vi "PicRead.vi"() -> ()   [LabVIEW 2012]
panel:
  out "二维图片":picture
  in  "path to JPEG file":path caption="JPEG文件路径"
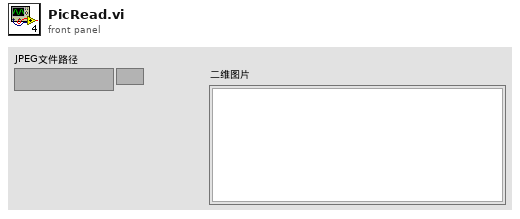
[diagram p1: front panel]
types:
  T1 = typedef "imagedata.ctl" = cluster{"image type":i32, "image depth":i32, "image":u8[], "mask":u8[], "colors":u32[], "Rectangle":cluster{"left":i16, "top":i16, "right":i16, "bottom":i16}}
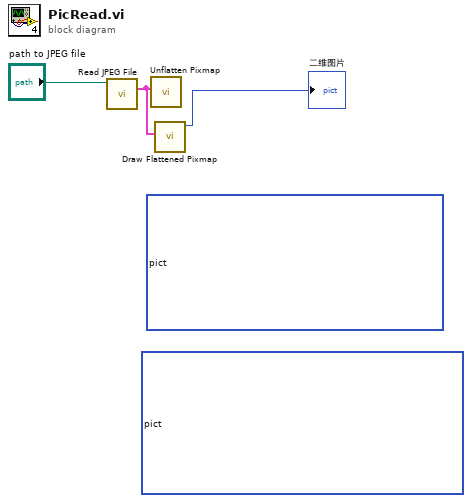
[diagram p0: block diagram]
diagram:
  (unwired) picture bytes[79491] ("二维图片")
  (unwired) picture bytes[79491] ("二维图片")
  n1 = call <vilib>:"Read JPEG File.vi"("path to JPEG file"="path to JPEG file") -> ("image data"=w2:T1)  [unwired: 8 in, 2 out]
  n2 = call <vilib>:"Unflatten Pixmap.vi"("image data"=w2) -> ()  [unwired: 4 in, 7 out]
  n3 = call <vilib>:"Draw Flattened Pixmap.vi"("image data"=w2) -> ("new picture"=→"二维图片":picture)  [unwired: 8 in]
